vi "Encode DCW Parameters.vi"(8 "ADD Parameters (in)":string, 9 "Scanner Settings In":T1={"Scan1"=1, "Scan2"=1, "Scan3"=1, "Scan4"=1, "Scan5"=1, "Scan6"=1, "Scan7"=1, "Scan8"=1, "Scan9"=1, "Scan10"=1, "Scan11"=1, "Scan12"=1, "Scan13"=1, "Scan14"=1, "Scan15"=1, "Scan16"=1} {"Scan16" scale=0.0..2.0; "Scan15" scale=0.0..2.0; "Scan14" scale=0.0..2.0; "Scan13" scale=0.0..2.0; "Scan12" scale=0.0..2.0; "Scan11" scale=0.0..2.0; "Scan10" scale=0.0..2.0; "Scan9" scale=0.0..2.0; "Scan8" scale=0.0..2.0; "Scan7" scale=0.0..2.0; "Scan6" scale=0.0..2.0; "Scan5" scale=0.0..2.0; "Scan4" scale=0.0..2.0; "Scan3" min=0 max=2 scale=0.0..2.0; "Scan2" min=0 max=2 scale=0.0..2.0; "Scan1" min=0 max=2 scale=0.0..2.0}, 10 "Internal Scanner Exists?":bool, 11 "DCW Test Parameters (in)":T2={"Voltage (0~6.0 KV)"=1.0, "High Limit(0.0~7500 uA)"=0.0, "Low Limit(0~7500 uA)"=0.0, "Ramp Up Time (0.1~999.9 seconds)"=0.4, "Dwell Time (0, 0.4~999.9 seconds)"=1.0, "Ramp Down Time (0, 1.0~999.9 seconds)"=0.0, "Charge LO (0.0~350uA)"=0.0, "Arc Sense (1~9)"=5, "Arc Detect (F: Off)"=FALSE, "Auto Charge LO (F: Off)"=FALSE, "Ramp-Hi (0.0~7500 uA)"=0.0} {"Ramp-Hi (0.0~7500 uA)" format="%.2f"; "Ramp Down Time (0, 1.0~999.9 seconds)" format="%.1f"; "Charge LO (0.0~350uA)" format="%.2f"; "Dwell Time (0, 0.4~999.9 seconds)" format="%.1f"; "Ramp Up Time (0.1~999.9 seconds)" format="%.1f"; "Low Limit(0~7500 uA)" format="%.1f"; "High Limit(0.0~7500 uA)" format="%.1f"; "Voltage (0~6.0 KV)" format="%.3f"}) -> (1 "DCW Test Parameters (out)":T2={"Voltage (0~6.0 KV)"=1.0, "High Limit(0.0~7500 uA)"=0.0, "Low Limit(0~7500 uA)"=0.0, "Ramp Up Time (0.1~999.9 seconds)"=0.4, "Dwell Time (0, 0.4~999.9 seconds)"=1.0, "Ramp Down Time (0, 1.0~999.9 seconds)"=0.0, "Charge LO (0.0~350uA)"=0.0, "Arc Sense (1~9)"=5, "Arc Detect (F: Off)"=FALSE, "Auto Charge LO (F: Off)"=FALSE, "Ramp-Hi (0.0~7500 uA)"=0.0} {"Ramp-Hi (0.0~7500 uA)" format="%.2f"; "Ramp Down Time (0, 1.0~999.9 seconds)" format="%.1f"; "Charge LO (0.0~350uA)" format="%.2f"; "Dwell Time (0, 0.4~999.9 seconds)" format="%.1f"; "Ramp Up Time (0.1~999.9 seconds)" format="%.1f"; "Low Limit(0~7500 uA)" format="%.1f"; "High Limit(0.0~7500 uA)" format="%.1f"}, 2 "Scanner Settings Out":T1={"Scan1"=1, "Scan2"=1, "Scan3"=1, "Scan4"=1, "Scan5"=1, "Scan6"=1, "Scan7"=1, "Scan8"=1, "Scan9"=1, "Scan10"=1, "Scan11"=1, "Scan12"=1, "Scan13"=1, "Scan14"=1, "Scan15"=1, "Scan16"=1} {"Scan16" scale=0.0..2.0; "Scan15" scale=0.0..2.0; "Scan14" scale=0.0..2.0; "Scan13" scale=0.0..2.0; "Scan12" scale=0.0..2.0; "Scan11" scale=0.0..2.0; "Scan10" scale=0.0..2.0; "Scan9" scale=0.0..2.0; "Scan8" scale=0.0..2.0; "Scan7" scale=0.0..2.0; "Scan6" scale=0.0..2.0; "Scan5" scale=0.0..2.0; "Scan4" scale=0.0..2.0; "Scan3" min=0 max=2 scale=0.0..2.0; "Scan2" min=0 max=2 scale=0.0..2.0; "Scan1" min=0 max=2 scale=0.0..2.0}, 3 "Add Parameters":string)   [LabVIEW 2016, in "eec EST 300.lvlib"]
uses:
  <instrlib>/eec EST 300/eec EST 300.lvlib
  <instrlib>/eec EST 300/Public/Configure/Steps/Low Level/DCW Test Parameters.ctl
  <instrlib>/eec EST 300/Public/Configure/Steps/Low Level/Scanner Settings.ctl
panel:
  # "On\nOff"
  # "On\nOff"
  # "On\nOff"
  # "On\nOff"
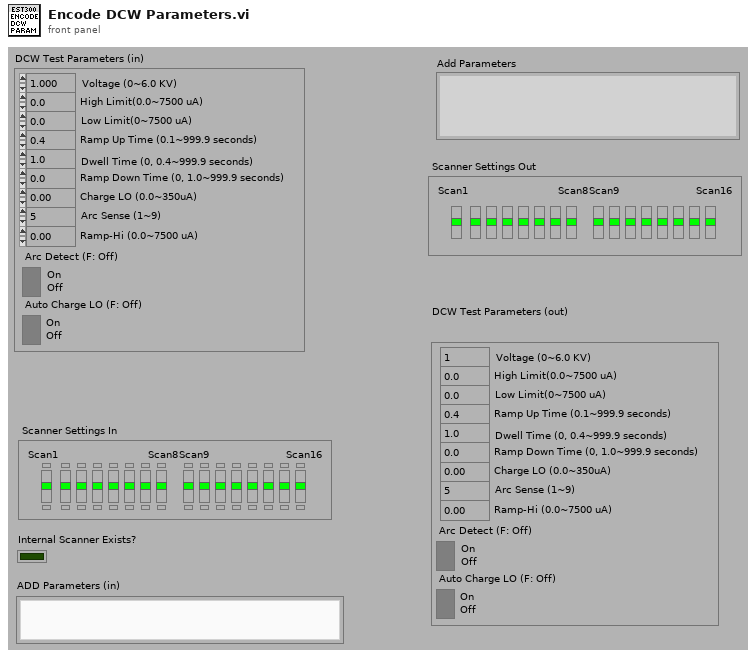
[diagram p1: front panel]
types:
  T1 = typedef "eec EST 300.lvlib/Scanner Settings.ctl" = cluster{"Scan1":i32, "Scan2":i32, "Scan3":i32, "Scan4":i32, "Scan5":i32, "Scan6":i32, "Scan7":i32, "Scan8":i32, "Scan9":i32, "Scan10":i32, "Scan11":i32, "Scan12":i32, "Scan13":i32, "Scan14":i32, "Scan15":i32, "Scan16":i32}
  T2 = typedef "eec EST 300.lvlib/DCW Test Parameters.ctl" = cluster{"Voltage (0~6.0 KV)":dbl, "High Limit(0.0~7500 uA)":dbl, "Low Limit(0~7500 uA)":dbl, "Ramp Up Time (0.1~999.9 seconds)":dbl, "Dwell Time (0, 0.4~999.9 seconds)":dbl, "Ramp Down Time (0, 1.0~999.9 seconds)":dbl, "Charge LO (0.0~350uA)":dbl, "Arc Sense (1~9)":i32, "Arc Detect (F: Off)":bool, "Auto Charge LO (F: Off)":bool, "Ramp-Hi (0.0~7500 uA)":dbl}
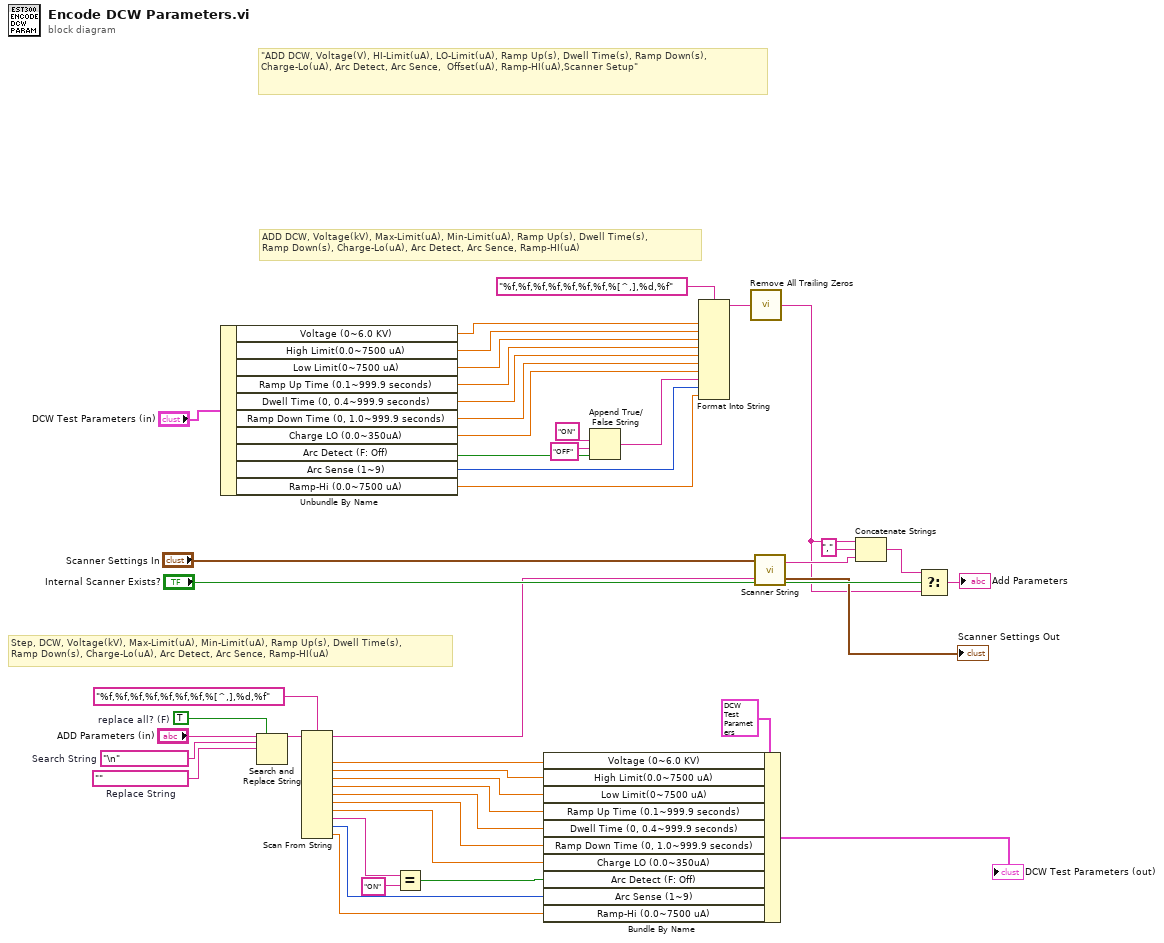
[diagram p0: block diagram]
diagram:
  w34 = TRUE  # replace all? (F)
  w35 = ""  # Replace String
  w36 = "\n"  # Search String
  # "ADD DCW, Voltage(kV), Max-Limit(uA), Min-Limit(uA), Ramp Up(s), Dwell Time(s), \nRamp Down(s), Charge-Lo(uA), Arc Detect, Arc Sence, Ramp-HI(uA)"
  # "Step, DCW, Voltage(kV), Max-Limit(uA), Min-Limit(uA), Ramp Up(s), Dwell Time(s), \nRamp Down(s), Charge-Lo(uA), Arc Detect, Arc Sence, Ramp-HI(uA)"
  # "\"ADD DCW, Voltage(V), HI-Limit(uA), LO-Limit(uA), Ramp Up(s), Dwell Time(s), Ramp Down(s), \nCharge-Lo(uA), Arc Detect, Arc Sence,  Offset(uA), Ramp-HI(uA),Scanner Setup\""
  n1 = Unbundle By Name("DCW Test Parameters (in)") -> ("Voltage (0~6.0 KV)"=w45:dbl, "High Limit(0.0~7500 uA)"=w29:dbl, "Low Limit(0~7500 uA)"=w44:dbl, "Ramp Up Time (0.1~999.9 seconds)"=w43:dbl, "Dwell Time (0, 0.4~999.9 seconds)"=w42:dbl, "Ramp Down Time (0, 1.0~999.9 seconds)"=w41:dbl, "Charge LO (0.0~350uA)"=w40:dbl, "Arc Detect (F: Off)"=w28:bool, "Arc Sense (1~9)"=w26:i32, "Ramp-Hi (0.0~7500 uA)"=w25:dbl)
  n2 = Search and Replace String(replace all?=w34, input string="ADD Parameters (in)", search string=w36, replace string=w35) -> (result string=w32:string)  [unwired: 4 in, 3 out]
  n3 = Scan From String(format string="%f,%f,%f,%f,%f,%f,%f,%[^,],%d,%f" ("Format String"), input string=w32) -> (remaining string=w19:string, output 1=w7:dbl, output 2=w6:dbl, output 3=w5:dbl, output 4=w4:dbl, output 5=w3:dbl, output 6=w2:dbl, output 7=w1:dbl, output 8=w12:string, output 9=w8:i32, output 10=w9:dbl)  [unwired: 12 in, 2 out]
  n4 = Equal?(x=w12, y="ON") -> (x = y?=w10:bool)
  n5 = Bundle By Name(cluster=T2 {"Voltage (0~6.0 KV)"=1.0, "High Limit(0.0~7500 uA)"=0.0, "Low Limit(0~7500 uA)"=0.0, "Ramp Up Time (0.1~999.9 seconds)"=0.4, "Dwell Time (0, 0.4~999.9 seconds)"=1.0, "Ramp Down Time (0, 1.0~999.9 seconds)"=0.0, "Charge LO (0.0~350uA)"=0.0, "Arc Sense (1~9)"=5, "Arc Detect (F: Off)"=FALSE, "Auto Charge LO (F: Off)"=FALSE, "Ramp-Hi (0.0~7500 uA)"=0.0} ("DCW Test Parameters (out) 2"), "Voltage (0~6.0 KV)"=w7, "High Limit(0.0~7500 uA)"=w6, "Low Limit(0~7500 uA)"=w5, "Ramp Up Time (0.1~999.9 seconds)"=w4, "Dwell Time (0, 0.4~999.9 seconds)"=w3, "Ramp Down Time (0, 1.0~999.9 seconds)"=w2, "Charge LO (0.0~350uA)"=w1, "Arc Detect (F: Off)"=w10, "Arc Sense (1~9)"=w8, "Ramp-Hi (0.0~7500 uA)"=w9) -> (→"DCW Test Parameters (out)":T2)
  n6 = Append True/False String(1:w28, 2:"OFF" ("false string"), 3:"ON" ("true string")) -> (0:w27:string)  [unwired: 1 in]
  n7 = Format Into String(format string="%f,%f,%f,%f,%f,%f,%f,%[^,],%d,%f" ("Format String"), w45, w29, w44, w43, w42, w41, w40, w27, w26, w25) -> (resulting string=w18:string)  [unwired: 2 in, 1 out]
  n8 = call <instrlib>:"Remove All Trailing Zeros.vi"("String in"=w18) -> ("String out"=w17:string)
  n9 = call <instrlib>:"Scanner String.vi"("Scanner String (in)"=w19, "Scanner Settings in"="Scanner Settings In") -> ("Scanner Settings out"=→"Scanner Settings Out":T1, "Scanner String (out)"=w20:string)
  n10 = Concatenate Strings(w17, "," ("Substring"), w20) -> (w37:string)
  n11 = Select(t=w37, s="Internal Scanner Exists?", f=w17) -> (s? t:f=→"Add Parameters":string)
